vi "setImage.vi"(8 "error in (no error)":errorcluster, 10 "Image Name":string="untitled", 11 "Stimulus in":refnum<class "Stimulus.lvclass">) -> (0 "error out":errorcluster, 3 "Stimulus out":refnum<class "Stimulus.lvclass">)   [LabVIEW 2013, in "Stimulus.lvclass"]
uses:
  Stimulus.lvclass
  Stimulus.lvclass/Stimulus.ctl
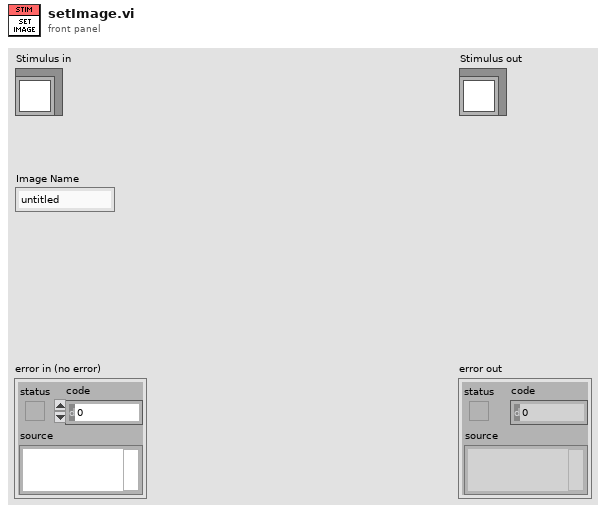
[diagram p1: front panel]
types:
  T1 = typedef "IMAQ Image.ctl" = refnum<image>
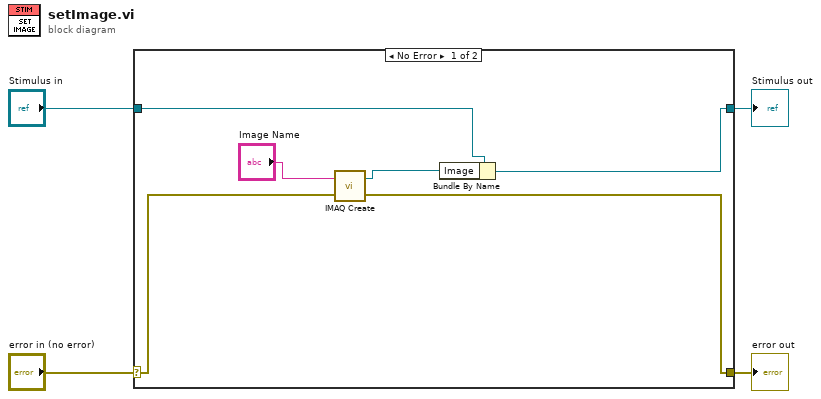
[diagram p0: block diagram]
diagram:
  n1 = case shown="No Error" "error in (no error)" {
    selector: "error in (no error)" -> [w7 w12]
    tunnel: [w6 w12] -> w3
    tunnel: [w9 w11] -> w1
    tunnel: "Stimulus in" -> [w10 w11]
    frame No Error {
      n2 = call "IMAQ Create"("Image Name"="Image Name", "error in (no error)"=w7) -> ("New Image"=w8:T1, "error out"=w6:errorcluster)  [unwired: 3 in]
      n3 = Bundle By Name(cluster=w10, "Image"=w8) -> (w9:refnum<class "Stimulus.lvclass">)
    }
    frame Error {
    }
  }
  "error out" <- w3
  "Stimulus out" <- w1
